vi "WPI_DashboardFormatPerf.vi"(9 "Right Camera Perf":cluster{"Bandwidth (Mbps)":dbl, "FPS":dbl}, 10 "Performance":cluster{"Bandwidth (Mbps)":dbl, "fps":dbl}, 11 "String in":refnum<vi>) -> ()   [LabVIEW 2025]
doc: "Format and display camera performance information from up to two cameras into a string indicator."
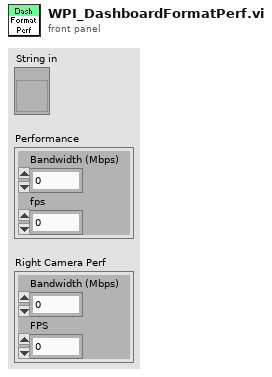
[diagram p1: front panel]
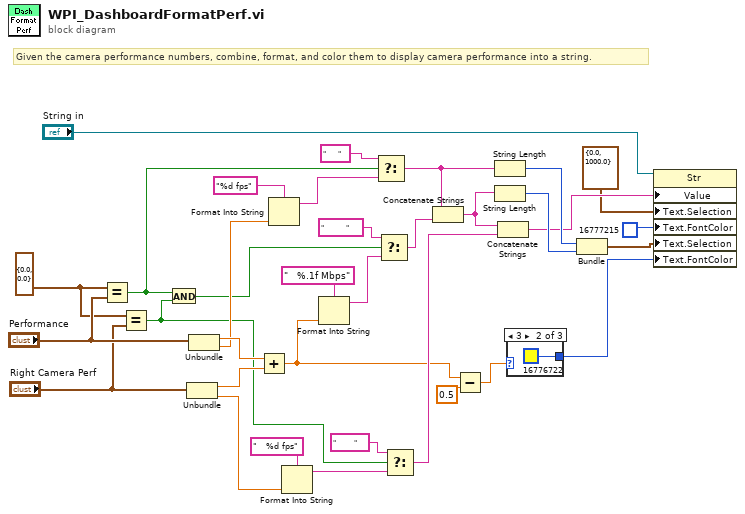
[diagram p0: block diagram]
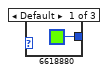
[diagram p2: hidden frame]
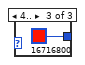
[diagram p3: hidden frame]
diagram:
  w18 = cluster{"Bandwidth (Mbps)":dbl, "fps":dbl} {"Bandwidth (Mbps)"=0.0, "fps"=0.0} ("Performance")
  # "Given the camera performance numbers, combine, format, and color them to display camera performance into a string."
  n1 = Equal?(x=w18, y="Performance") -> (x = y?=w13:bool)
  n2 = Equal?(x=w18, y="Right Camera Perf") -> (x = y?=w12:bool)
  n3 = And(x=w13, y=w12) -> (x .and. y?=w8:bool)
  n4 = Unbundle("Right Camera Perf") -> ("Bandwidth (Mbps)"=w33:dbl, "FPS"=w28:dbl)
  n5 = Unbundle("Performance") -> ("Bandwidth (Mbps)"=w34:dbl, "fps"=w31:dbl)
  n6 = Add(x=w34, y=w33) -> (x+y=w2:dbl)
  n7 = Format Into String(format string="%d fps", w31) -> (resulting string=w7:string)  [unwired: 2 in, 1 out]
  n8 = Format Into String(format string="   %d fps", w28) -> (resulting string=w15:string)  [unwired: 2 in, 1 out]
  n9 = Format Into String(format string="   %.1f Mbps", w2) -> (resulting string=w9:string)  [unwired: 2 in, 1 out]
  n10 = Select(t="      " ("format string"), s=w13, f=w7) -> (s? t:f=w6:string)
  n11 = Select(t="           " ("format string"), s=w8, f=w9) -> (s? t:f=w10:string)
  n12 = Select(t="         " ("format string"), s=w12, f=w15) -> (s? t:f=w14:string)
  n13 = Concatenate Strings(w6, w10) -> (w22:string)
  n14 = Subtract(x=w2, y=0.5 ("Bandwidth (Mbps)")) -> (x-y=w1:dbl)
  n15 = String Length(string=w6) -> (length=w26:i32)
  n16 = String Length(string=w22) -> (length=w25:i32)
  n17 = Concatenate Strings(w22, w14) -> (w21:string)
  n18 = case shown="3" w1 {
    tunnel: [u32 6618880 ("Color Box") u32 16776722 ("Color Box") u32 16716800 ("Color Box")] -> w23
    frame Default {
    }
    frame 3 {
    }
    frame 4.. {
    }
  }
  n19 = Bundle(w26, w25) -> (w24:cluster{i32, i32})  [unwired: 1 in]
  n20 = property class="Str"(reference="String in", "Value"=w21, "Text.Selection"=cluster{"Bandwidth (Mbps)":dbl, "fps":dbl} {"Bandwidth (Mbps)"=0.0, "fps"=1000.0} ("Performance"), "Text.FontColor"=u32 16777215 ("Color Box"), "Text.Selection"=w24, "Text.FontColor"=w23) -> ()  [unwired: 1 in, 2 out]
